vi "Insert Below.vi"(8 "error in (no error)":errorcluster, 9 "Item Tag":string, 10 "Tree Refnum":refnum<vi>, 11 "Tree Click Interpreter in":refnum<class "Tree Click Interpreter.lvclass">) -> (0 "error out":errorcluster, 1 "Insertion Index":i32, 2 "Parent ID":string, 3 "Tree Click Interpreter out":refnum<class "Tree Click Interpreter.lvclass">)   [LabVIEW 2017, in "Tree Click Interpreter.lvclass"]
uses:
  Tree Click Interpreter.lvclass
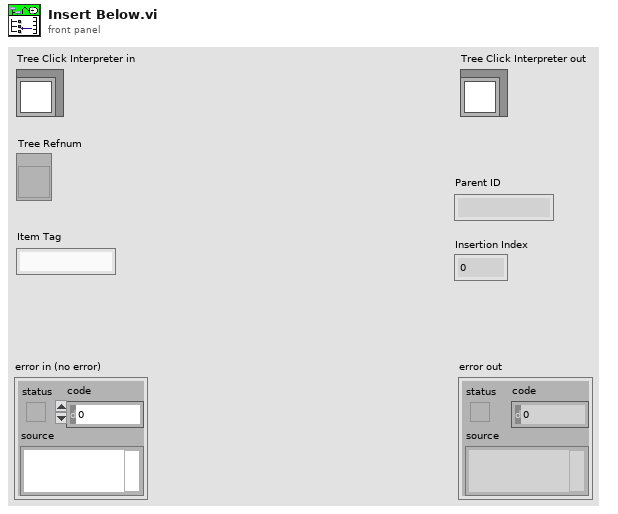
[diagram p1: front panel]
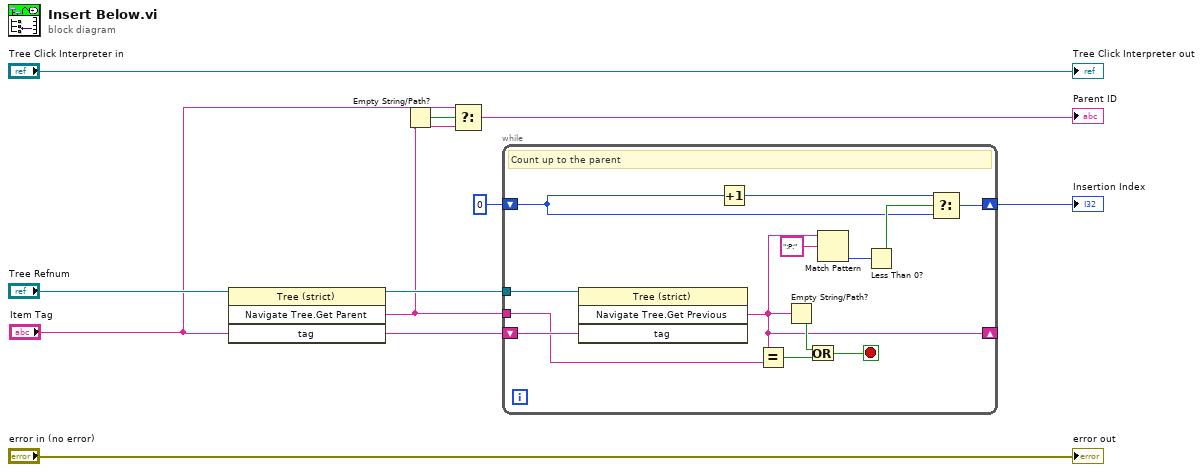
[diagram p0: block diagram]
diagram:
  n1 = invoke class="Tree (strict)" method="Navigate Tree.Get Parent"(reference="Tree Refnum", "tag"="Item Tag") -> (reference out=w7:refnum<vi>, "Navigate Tree:Get Parent"=w5:string)  [unwired: 2 in, 2 out]
  n2 = Empty String/Path?(string/path=w5) -> (empty?=w6:bool)
  n3 = Select(t="Item Tag", s=w6, f=w5) -> (s? t:f=→"Parent ID":string)
  n4 = while {
    shift-right: [w11] -> w1
    shift-left: 0 -> [w13]
    tunnel: w7 -> [w23]
    tunnel: w5 -> [w21]
    shift-right: [w17] -> _
    shift-left: "Item Tag" -> [w22]
    stop <- w18 stop-if-true
    # "Count up to the parent"
    n5 = invoke class="Tree (strict)" method="Navigate Tree.Get Previous"(reference=w23, "tag"=w22) -> ("Navigate Tree:Get Previous"=w17:string)  [unwired: 2 in, 3 out]
    n6 = Increment(x=w13) -> (x+1=w12:i32)
    n7 = Equal?(x=w17, y=w21) -> (x = y?=w20:bool)
    n8 = Empty String/Path?(string/path=w17) -> (empty?=w19:bool)
    n9 = Or(x=w19, y=w20) -> (x .or. y?=w18:bool)
    n10 = Match Pattern(string=w17, regular expression=":P:") -> (offset past match=w15:i32)  [unwired: 1 in, 3 out]
    n11 = Less Than 0?(x=w15) -> (x < 0?=w14:bool)
    n12 = Select(t=w12, s=w14, f=w13) -> (s? t:f=w11:i32)
  }
  "Insertion Index" <- w1
  "error out" <- "error in (no error)"
  "Tree Click Interpreter out" <- "Tree Click Interpreter in"
